vi "run.vi"(8 "error in (no error)":errorcluster, 10 "Log in":refnum<class "Log.lvclass">, 11 "AndorController in":refnum<class "AndorController.lvclass">) -> (0 "error out":errorcluster, 2 "Log out":refnum<class "Log.lvclass">, 3 "AndorController out":refnum<class "AndorController.lvclass">)   [LabVIEW 2011, in "Hardware.lvlib" / "Channels.lvlib" / "AndorController.lvclass"]
uses:
  AndorController.lvclass
  Tools/Log.lvclass
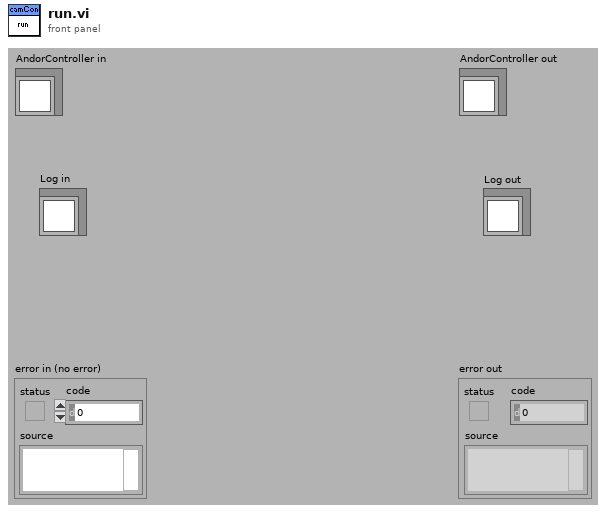
[diagram p1: front panel]
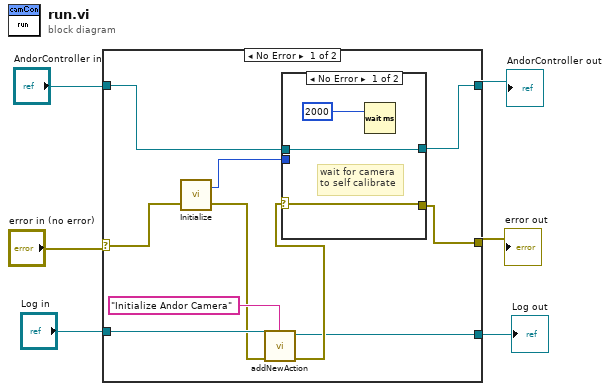
[diagram p0: block diagram]
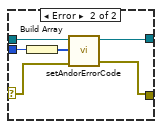
[diagram p2: hidden frame]
diagram:
  n1 = case shown="No Error" "error in (no error)" {
    selector: "error in (no error)" -> [w16 w26]
    tunnel: "AndorController in" -> [w15 w27]
    tunnel: [w14 w27] -> w4
    tunnel: [w12 w26] -> w3
    tunnel: "Log in" -> [w11 _]
    tunnel: [w7 _] -> w1
    frame No Error {
      n2 = call <userlib>:"Initialize.vi"("error in (no error)"=w16) -> ("error out"=w9:errorcluster, "DLL error code"=w13:u32)  [unwired: 1 in]
      n3 = call-dynamic "addNewAction.vi"("error in (no error)"=w9, "newAction"="Initialize Andor Camera", "Log in"=w11) -> ("error out"=w8:errorcluster, "Log out"=w7:refnum<class "Log.lvclass">)  [unwired: 7 in]
      n4 = case shown="No Error" w8 {
        selector: w8 -> [w18 w23]
        tunnel: w15 -> [w17 w25]
        tunnel: [w17 w24] -> w14
        tunnel: w13 -> [_ w21]
        tunnel: [w18 w22] -> w12
        frame No Error {
          # "wait for camera\nto self calibrate"
          n5 = Wait (ms)(milliseconds to wait=2000) -> ()  [unwired: 1 out]
        }
        frame Error {
          n6 = Build Array(w21) -> (w20:u32[])
          n7 = call "setAndorErrorCode.vi"("error in (no error)"=w23, "Andor Error Codes"=w20, "AndorController.lvclass in"=w25) -> ("error out"=w22:errorcluster, "AndorController.lvclass out"=w24:refnum<class "AndorController.lvclass">)  [unwired: 7 in]
        }
      }
    }
    frame Error {
    }
  }
  "error out" <- w3
  "AndorController out" <- w4
  "Log out" <- w1
